vi "RichToFlatcif_manager_QuerySettings.vi"(5 "OutputClusterType":T1, 11 "InputCluster":T2) -> (3 "OutputCluster":T1)   [LabVIEW 2021, in "CIF_Manager_client.lvlib"]
uses:
  CIF_Manager_client.lvlib
  cif_manager_QuerySettings.ctl
  cif_manager_QuerySettings_Flat.ctl
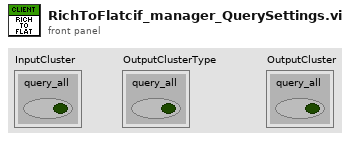
[diagram p1: front panel]
types:
  T1 = typedef "CIF_Manager_client.lvlib/cif_manager_QuerySettings_Flat.ctl" = cluster{"query_all":bool}
  T2 = typedef "CIF_Manager_client.lvlib/cif_manager_QuerySettings.ctl" = cluster{"query_all":bool}
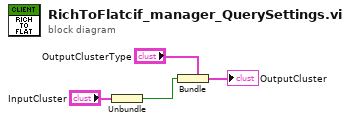
[diagram p0: block diagram]
diagram:
  n1 = Unbundle "Unbundle"("InputCluster") -> ("query_all"=w1:bool)
  n2 = Bundle "Bundle"(cluster="OutputClusterType", "query_all"=w1) -> (→"OutputCluster":T1)
